vi "pidGrapher.vi"(8 "targetCurrent":dbl, 9 "valueCurrent":dbl, 10 "timeCurrent":dbl, 11 "n":i32) -> (3 "XY Graph":cluster{dbl[], dbl[]}[](graph))   [LabVIEW 2012]
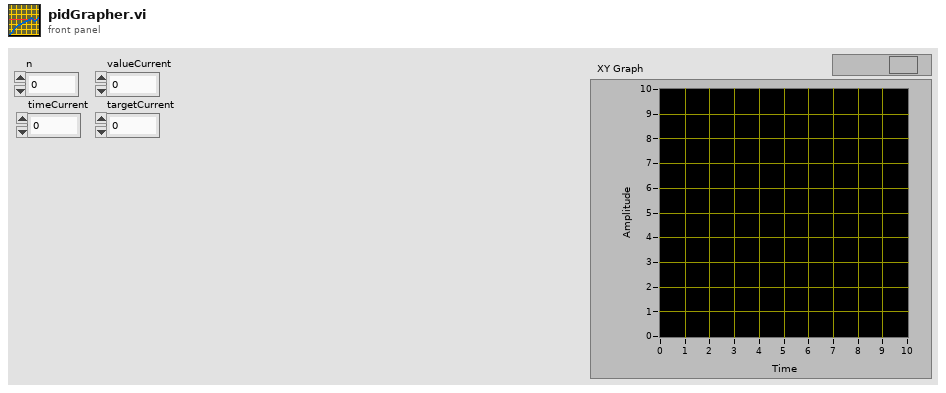
[diagram p1: front panel]
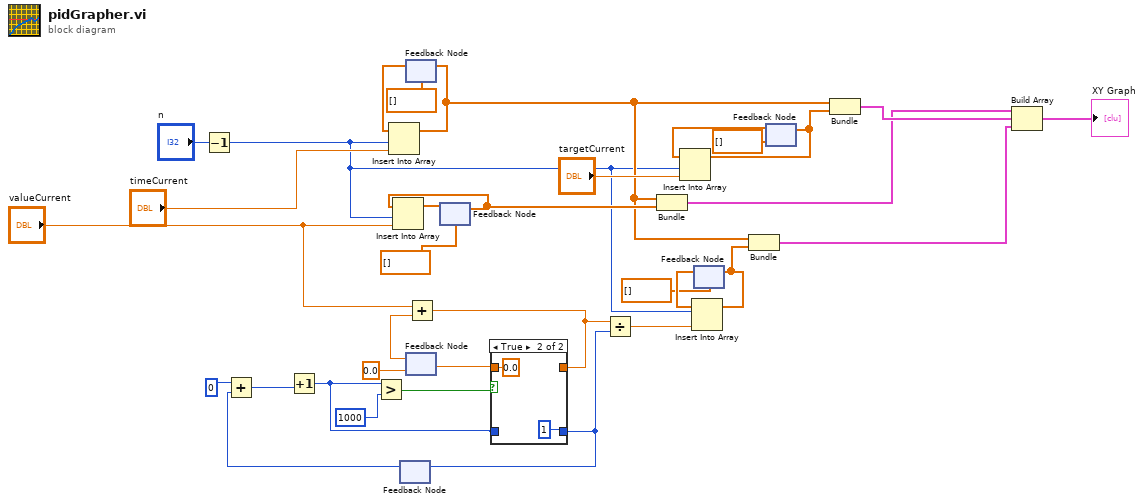
[diagram p0: block diagram]
diagram:
  n1 = Decrement(x="n") -> (x-1=w4:i32)
  n2 = feedback #1() -> (w9:i32)  [unwired: 1 in]
  n3 = Add(x=0, y=w9) -> (x+y=w10:i32)
  n4 = Increment(x=w10) -> (x+1=w15:i32)
  n5 = Greater?(x=w15, y=1000) -> (0:w16:bool)
  n6 = feedback #2(dbl[] []) -> (w32:dbl[])
  n7 = Insert Into Array(array=w32, index=w4, new element="timeCurrent") -> (w20:dbl[])
  n8 = feedback-in #2(w20) -> ()
  n9 = feedback #3(0.0) -> (w13:dbl)
  n10 = Add(x="valueCurrent", y=w13) -> (x+y=w8:dbl)
  n11 = feedback #4(dbl[] []) -> (w21:dbl[])
  n12 = Insert Into Array(array=w21, index=w4, new element="valueCurrent") -> (w30:dbl[])
  n13 = feedback-in #4(w30) -> ()
  n14 = case shown="True" w16 {
    tunnel: w8 -> [w35 _]
    tunnel: w15 -> [w34 _]
    tunnel: [w35 0.0] -> w14
    tunnel: [w34 1] -> w7
    frame False {
    }
    frame True {
    }
  }
  n15 = feedback-in #1(w7) -> ()
  n16 = feedback-in #3(w14) -> ()
  n17 = Divide(x=w8, y=w7) -> (x/y=w6:dbl)
  n18 = Bundle(w20, w21) -> (w22:cluster{dbl[], dbl[]})  [unwired: 1 in]
  n19 = feedback #5(dbl[] []) -> (w3:dbl[])
  n20 = Insert Into Array(array=w3, index=w4, new element=w6) -> (w1:dbl[])
  n21 = feedback-in #5(w1) -> ()
  n22 = Bundle(w20, w1) -> (w19:cluster{dbl[], dbl[]})  [unwired: 1 in]
  n23 = feedback #6(dbl[] []) -> (w27:dbl[])
  n24 = Insert Into Array(array=w27, index=w4, new element="targetCurrent") -> (w24:dbl[])
  n25 = feedback-in #6(w24) -> ()
  n26 = Bundle(w20, w24) -> (w23:cluster{dbl[], dbl[]})  [unwired: 1 in]
  n27 = Build Array(w22, w23, w19) -> (→"XY Graph":cluster{dbl[], dbl[]}[])
